vi "lv-getBuildSpecTag.vi"(8 "error in (no error)":errorcluster, 10 "Tag name":string, 11 "Project refs":T1={"LabVIEW Project Path"=path "C:/Users/admin/Desktop/Source/Waveform-Processing-Custom-Device.lvproj", "Project refnum"=refnum, "Build spec refnum"=refnum}) -> (0 "error out":errorcluster, 3 "Project refs out":T1={"LabVIEW Project Path"=path "C:/Users/admin/Desktop/Source/Waveform-Processing-Custom-Device.lvproj", "Project refnum"=refnum, "Build spec refnum"=refnum}, 9 "Tag value":string)   [LabVIEW 2014, in "lv-build-library.lvlib"]
uses:
  lv-build-library.lvlib
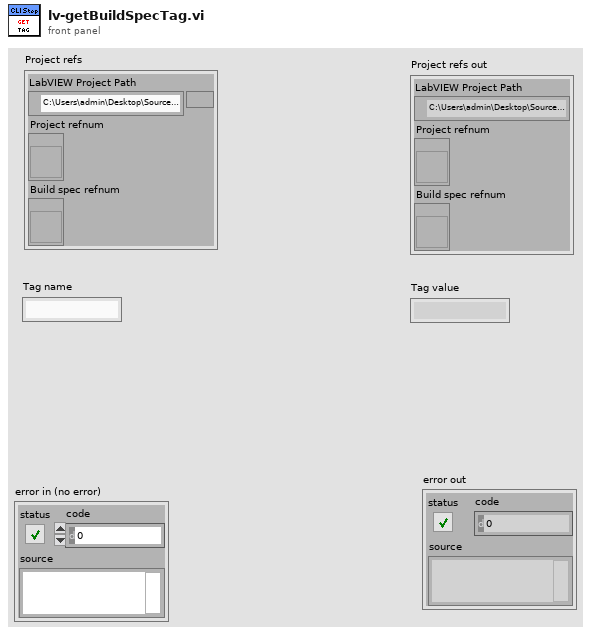
[diagram p1: front panel]
types:
  T1 = cluster{"LabVIEW Project Path":path, "Project refnum":refnum<vi>, "Build spec refnum":refnum<vi>}
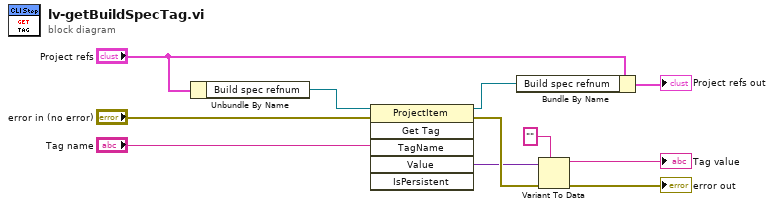
[diagram p0: block diagram]
diagram:
  n1 = Unbundle By Name("Project refs") -> ("Build spec refnum"=w9:refnum<vi>)
  n2 = invoke class="ProjectItem" method="Get Tag"(reference=w9, error in="error in (no error)", "TagName"="Tag name") -> (reference out=w7:refnum<vi>, error out=w5:errorcluster, "Value"=w4:variant)  [unwired: 3 in, 3 out]
  n3 = Bundle By Name(cluster="Project refs", "Build spec refnum"=w7) -> (→"Project refs out":T1)
  n4 = Variant To Data(error in=w5, type="", Variant=w4) -> (data=→"Tag value":string, error out=→"error out":errorcluster)
